vi "Send message (SubVI).vi"(4 "lockout_key":string, 5 "input json string":string, 6 "retcode":u16, 7 "msgop":i32, 8 "error in (no error)":errorcluster, 9 "msgtype":i32, 10 "routing key":string, 11 "Exchange in":refnum<class "Exchange.lvclass">) -> (0 "error out":errorcluster, 3 "Exchange out":refnum<class "Exchange.lvclass">)   [LabVIEW 2016]
uses:
  <vilib>/Distrio/LabbitMQ/Exchange/Exchange.lvclass
  C:/Program Files (x86)/National Instruments/LabVIEW 2016/vi.lib/Distrio/LabbitMQ/RabbitMQ.Client.dll
  Program Files (x86)/National Instruments/LabVIEW 2016/vi.lib/Distrio/LabbitMQ/RabbitMQ.Client.dll
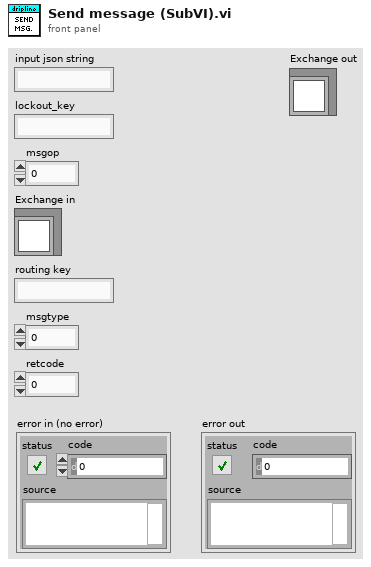
[diagram p1: front panel]
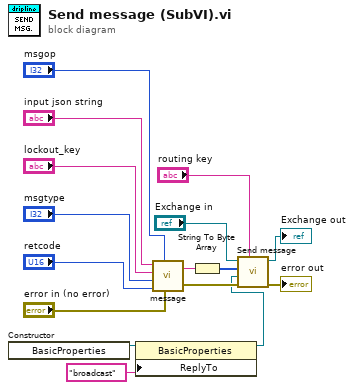
[diagram p0: block diagram]
diagram:
  n1 = constructor class="BasicProperties"() -> (reference out=w1:refnum<k24>)  [unwired: 3 in, 2 out]
  n2 = property class="BasicProperties"(reference=w1, "ReplyTo"="broadcast") -> (reference out=w2:refnum<k24>)  [unwired: 1 in, 1 out]
  n3 = call "message.vi"("error in (no error)"="error in (no error)", "msgop"="msgop", "retcode"="retcode", "msgtype"="msgtype", "lockout_key"="lockout_key", "input json string"="input json string") -> ("error out"=w15:errorcluster, "body"=w9:string)
  n4 = String To Byte Array(string=w9) -> (unsigned byte array=w10:u8[])
  n5 = call <vilib>:"Send message.vi"("routing key"="routing key", "error in (no error)"=w15, "MessageProperties"=w2, "body"=w10, "Exchange in"="Exchange in") -> ("error out"=→"error out":errorcluster, "Exchange out"=→"Exchange out":refnum<class "Exchange.lvclass">)  [unwired: 5 in]
